vi "EnableDisableCells.vi"(6 "Cell Position":T1, 7 "Item Name or Tag":string, 8 "error in (no error)":errorcluster, 9 "Col Array Ref in":refnum<vi>, 10 "Table CtlRef in":refnum<vi>, 11 "MenuDisableCol in":refnum<class "MenuDisableCol.lvclass">) -> (0 "error out":errorcluster, 1 "Col Array Ref out":refnum<vi>, 2 "Table CtlRef out":refnum<vi>, 3 "MenuDisableCol out":refnum<class "MenuDisableCol.lvclass">)   [LabVIEW 2013, in "MenuDisableCol.lvclass"]
uses:
  MenuDisableCol.lvclass
  <vilib>/Utility/miscctls.llb/LVRowAndColumnTypeDef.ctl
  MenuDisableCol.lvclass/MenuDisableCol.ctl
  Column/Column.lvclass
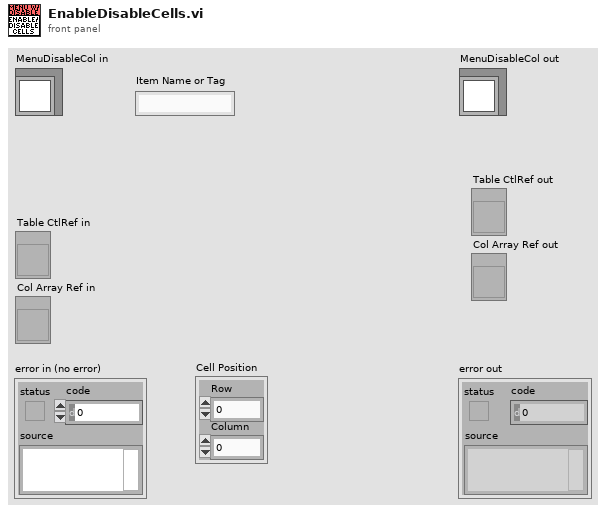
[diagram p1: front panel]
types:
  T1 = typedef "LVRowAndColumnTypeDef.ctl" = cluster{"Row":i32, "Column":i32}
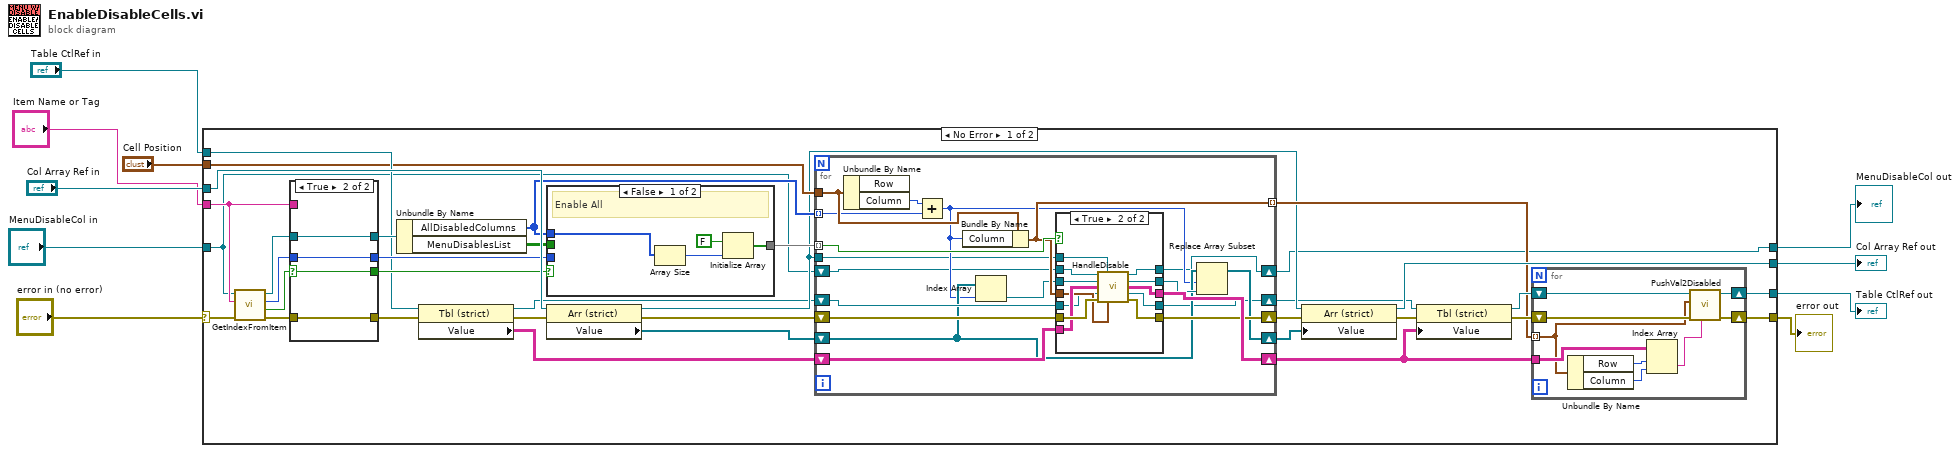
[diagram p0: block diagram]
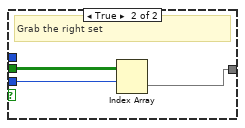
[diagram p2: hidden frame]
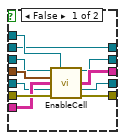
[diagram p3: hidden frame]
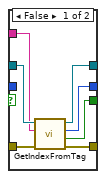
[diagram p4: hidden frame]
diagram:
  n1 = case shown="No Error" "error in (no error)" {
    selector: "error in (no error)" -> [w39 w118]
    tunnel: [w20 w118] -> w9
    tunnel: [w13 w117] -> w7
    tunnel: "MenuDisableCol in" -> [w14 w117]
    tunnel: "Table CtlRef in" -> [w27 w116]
    tunnel: [w21 w116] -> w5
    tunnel: "Col Array Ref in" -> [w38 w115]
    tunnel: [w31 w115] -> w3
    tunnel: "Cell Position" -> [w16 _]
    tunnel: "Item Name or Tag" -> [w43 _]
    frame No Error {
      n2 = call-dynamic "GetIndexFromItem.vi"("error in (no error)"=w39, "Item Name"=w43, "MenuCol in"=w14) -> ("error out"=w42:errorcluster, "Item Exists"=w45:bool, "Item Index"=w44:i32, "MenuCol out"=w41:refnum<class "MenuDisableCol.lvclass">)  [unwired: 5 in]
      n3 = case shown="True" w45 {
        selector: w45 -> [_ w113]
        tunnel: w44 -> [_ w112]
        tunnel: w43 -> [w104 _]
        tunnel: w42 -> [w110 w114]
        tunnel: [w109 w114] -> w25
        tunnel: [w108 w112] -> w35
        tunnel: [w107 w113] -> w37
        tunnel: [w106 w111] -> w40
        tunnel: w41 -> [w105 w111]
        frame False {
          n4 = call-dynamic "GetIndexFromTag.vi"("error in (no error)"=w110, "ItemTag"=w104, "MenuCol in"=w105) -> ("error out"=w109:errorcluster, "Item Exists"=w107:bool, "Item Index"=w108:i32, "MenuCol out"=w106:refnum<class "MenuDisableCol.lvclass">)  [unwired: 5 in]
        }
        frame True {
        }
      }
      n5 = Unbundle By Name(w40) -> ("AllDisabledColumns"=w23:i32[], "MenuDisablesList"=w36:bool[][])
      n6 = property class="Tbl (strict)"(reference=w27, error in=w25) -> (reference out=w12:refnum<vi>, error out=w24:errorcluster, "Value"=w26:string[][])
      n7 = case shown="False" w37 {
        tunnel: w36 -> [_ w61]
        tunnel: w35 -> [_ w60]
        tunnel: [w55 w59] -> w34
        tunnel: w23 -> [w56 _]
        frame False {
          # "Enable All"
          n8 = Array Size(array=w56) -> (size(s)=w57:i32)
          n9 = Initialize Array(FALSE, w57) -> (w55:bool[])
        }
        frame True {
          # "Grab the right set"
          n10 = Index Array(array=w61, index (row)=w60) -> (element=w59:bool[])  [unwired: 1 in]
        }
      }
      n11 = property class="Arr (strict)"(reference=w38, error in=w24) -> (reference out=w15:refnum<vi>, error out=w32:errorcluster, "Value"=w33:refnum<class "Column.lvclass">[])
      n12 = for {
        tunnel: w23 -> [w78] mode=indexing
        tunnel: w34 -> [w76] mode=indexing
        shift-right: [w67] -> w30
        shift-left: w33 -> [w68]
        shift-right: [w73] -> w29
        shift-left: w32 -> [w77]
        shift-right: [w74] -> w18
        shift-left: w26 -> [w72]
        tunnel: [w75] -> w17 mode=indexing
        tunnel: w16 -> [w80]
        tunnel: w15 -> [w65]
        shift-right: [w63] -> w13
        shift-left: w14 -> [w64]
        shift-right: [w62] -> w11
        shift-left: w12 -> [w71]
        n13 = Unbundle By Name(w80) -> ("Column"=w79:i32)  [unwired: 1 out]
        n14 = Add(x=w79, y=w78) -> (x+y=w66:i32)
        n15 = Bundle By Name(cluster=w80, "Column"=w66) -> (w75:T1)
        n16 = Index Array(array=w68, index=w66) -> (element=w70:refnum<class "Column.lvclass">)
        n17 = case shown="True" w76 {
          tunnel: w77 -> [w91 w103]
          tunnel: w75 -> [w90 w97]
          tunnel: [w89 w100] -> w74
          tunnel: [w88 w101] -> w73
          tunnel: [w87 w95] -> w69
          tunnel: w70 -> [w84 w96]
          tunnel: w72 -> [w86 w102]
          tunnel: w71 -> [w85 w93]
          tunnel: w65 -> [w83 w94]
          tunnel: w64 -> [w82 w99]
          tunnel: [w82 w98] -> w63
          tunnel: [w81 w92] -> w62
          frame False {
            n18 = call-dynamic "EnableCell.vi"("Column in"=w84, "Col Array Ref in"=w83, "Cell Position"=w90, "Table Data in"=w86, "Table CtlRef In"=w85, "error in (no error)"=w91) -> ("Column out"=w87:refnum<class "Column.lvclass">, "Table Data out"=w89:string[][], "Table CtlRef Out"=w81:refnum<vi>, "error out"=w88:errorcluster)  [unwired: 5 in, 1 out]
          }
          frame True {
            n19 = call-dynamic "HandleDisable.vi"("MenuDisableCol in"=w99, "Col Array Ref in"=w94, "ToDisable in"=w96, "Table Data in"=w102, "Table CtlRef in"=w93, "error in (no error)"=w103, "Cell Position"=w97) -> ("MenuDisableCol out"=w98:refnum<class "MenuDisableCol.lvclass">, "ToDisable out"=w95:refnum<class "Column.lvclass">, "Table Data out"=w100:string[][], "Table CtlRef Out"=w92:refnum<vi>, "error out"=w101:errorcluster)  [unwired: 4 in]
          }
        }
        n20 = Replace Array Subset(array=w68, new element=w69, index=w66) -> (w67:refnum<class "Column.lvclass">[])
      }
      n21 = property class="Arr (strict)"(reference=w15, error in=w29, "Value"=w30) -> (reference out=w31:refnum<vi>, error out=w28:errorcluster)
      n22 = property class="Tbl (strict)"(reference=w11, error in=w28, "Value"=w18) -> (reference out=w22:refnum<vi>, error out=w19:errorcluster)
      n23 = for {
        shift-right: [w53] -> w21
        shift-left: w22 -> [w54]
        shift-right: [w52] -> w20
        shift-left: w19 -> [w51]
        tunnel: w18 -> [w50]
        tunnel: w17 -> [w46] mode=indexing
        n24 = Unbundle By Name(w46) -> ("Row"=w48:i32, "Column"=w47:i32)
        n25 = Index Array(array=w50, index (row)=w48, index (col)=w47) -> (element=w49:string)
        n26 = call "PushVal2Disabled.vi"("Value"=w49, "error in (no error)"=w51, "Cell Position"=w46, "Table CtlRef In"=w54) -> ("error out"=w52:errorcluster, "Table CtlRef Out"=w53:refnum<vi>)  [unwired: 5 in, 1 out]
      }
    }
    frame Error {
    }
  }
  "error out" <- w9
  "MenuDisableCol out" <- w7
  "Table CtlRef out" <- w5
  "Col Array Ref out" <- w3
